vi "ValidateInputs.vi"(8 "error in (no error)":errorcluster, 11 "DiscoverTestCases in":refnum<class "DiscoverTestCases.lvclass">) -> (0 "error out":errorcluster, 3 "DiscoverTestCases out":refnum<class "DiscoverTestCases.lvclass">)   [LabVIEW 2027, in "DiscoverTestCases.lvclass"]
uses:
  DiscoverTestCases.lvclass
  DiscoverTestCases.lvclass/DiscoverTestCases.ctl
  <nishared>/LabVIEW CLI/Operations/Utilities/OperationErrorType.ctl
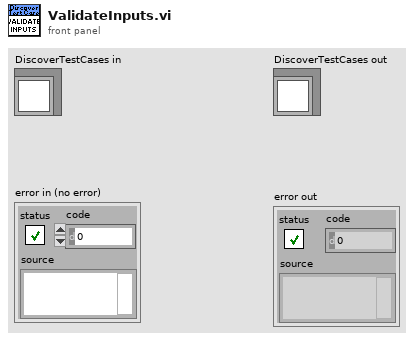
[diagram p1: front panel]
types:
  T1 = typedef "OperationErrorType.ctl" = enum16{"RequiredArgumentMissing", "UnknownArguments", "LoggerSetMultipleTimes", "OperationBrokenError"}
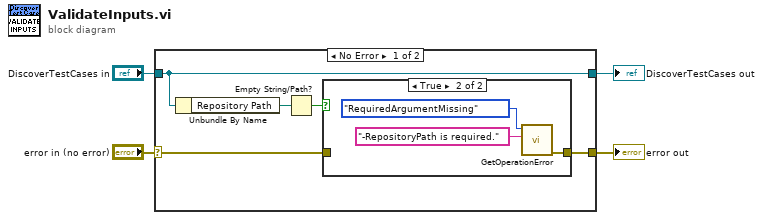
[diagram p0: block diagram]
diagram:
  n1 = case shown="No Error" "error in (no error)" {
    selector: "error in (no error)" -> [w7 w15]
    tunnel: [w6 w15] -> w4
    tunnel: "DiscoverTestCases in" -> [w5 w14]
    tunnel: [w5 w14] -> w1
    frame No Error {
      n2 = Unbundle By Name(w5) -> ("Repository Path"=w9:path)
      n3 = Empty String/Path?(string/path=w9) -> (empty?=w8:bool)
      n4 = case shown="True" w8 {
        tunnel: [w10 w13] -> w6
        tunnel: w7 -> [w10 _]
        frame False {
        }
        frame True {
          n5 = call <nishared>:"GetOperationError.vi"("Additional Information"="-RepositoryPath is required.", "Operation Error Type"=OperationErrorType."RequiredArgumentMissing") -> ("error out"=w13:errorcluster)  [unwired: 9 in]
        }
      }
    }
    frame Error {
    }
  }
  "DiscoverTestCases out" <- w1
  "error out" <- w4
